vi "NodeMenuSelection.vi"(8 "error in (no error)":errorcluster, 9 "Item Path in":string, 10 "Menu Path in":string, 11 "xceRootNode in":refnum<class "xceRootNode.lvclass">) -> (0 "error out":errorcluster, 1 "Item Path out":string, 2 "Menu Path out":string, 3 "xceRootNode out":refnum<class "xceRootNode.lvclass">)   [LabVIEW 2013, in "xceRootNode.lvclass"]
doc: "Determines the action that must be performed based on the users tree control menu selection."
uses:
  xceRootNode.lvclass
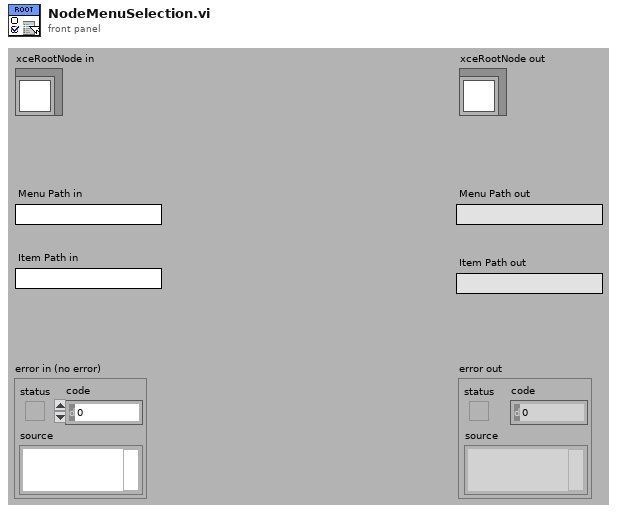
[diagram p1: front panel]
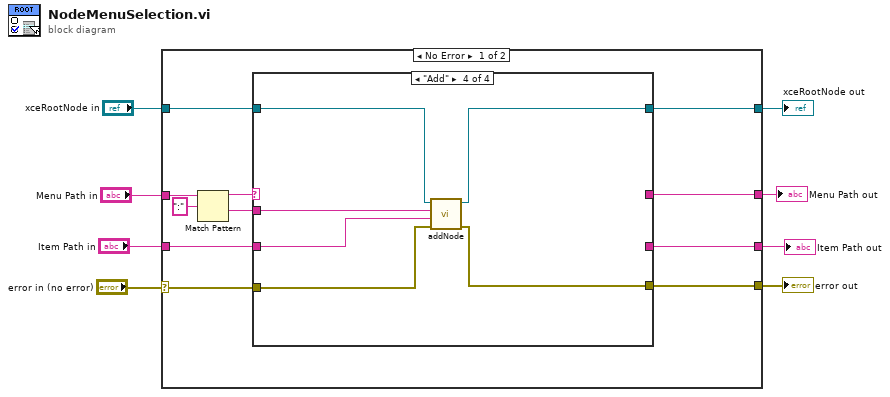
[diagram p0: block diagram]
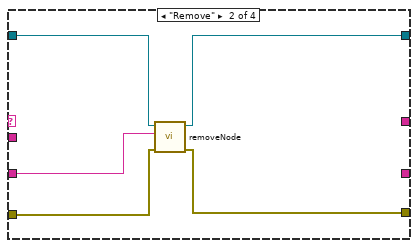
[diagram p3: hidden frame]
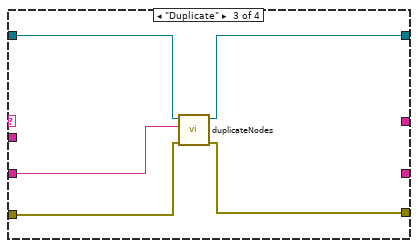
[diagram p4: hidden frame]
diagram:
  n1 = case shown="No Error" "error in (no error)" {
    selector: "error in (no error)" -> [w14 w41]
    tunnel: [w13 w41] -> w7
    tunnel: [w18 w40] -> w5
    tunnel: "xceRootNode in" -> [w19 w40]
    tunnel: "Menu Path in" -> [w12 _]
    tunnel: "Item Path in" -> [w17 _]
    tunnel: [w16 _] -> w2
    tunnel: [w15 _] -> w1
    frame No Error {
      n2 = Match Pattern(string=w12, regular expression=":") -> (before substring=w10:string, after substring=w9:string)  [unwired: 1 in, 2 out]
      n3 = case shown="\"Add\"" w10 {
        selector: w10 -> [w23 _ _ _]
        tunnel: w19 -> [w21 w28 w33 w39]
        tunnel: [w21 w27 w32 w38] -> w18
        tunnel: w17 -> [w22 w26 w31 w34]
        tunnel: [w23 _ _ _] -> w16
        tunnel: [w22 _ _ _] -> w15
        tunnel: w14 -> [w20 w25 w30 w36]
        tunnel: [w20 w24 w29 w35] -> w13
        tunnel: w9 -> [_ _ _ w37]
        frame "", Default {
        }
        frame "Remove" {
          n4 = call "removeNode.vi"("error in (no error)"=w25, "Node Path"=w26, "xceRootNode in"=w28) -> ("error out"=w24:errorcluster, "xceRootNode out"=w27:refnum<class "xceRootNode.lvclass">)  [unwired: 7 in]
        }
        frame "Duplicate" {
          n5 = call "duplicateNodes.vi"("error in (no error)"=w30, "Node Path"=w31, "xceRootNode in"=w33) -> ("error out"=w29:errorcluster, "xceRootNode out"=w32:refnum<class "xceRootNode.lvclass">)  [unwired: 7 in]
        }
        frame "Add" {
          n6 = call "addNode.vi"("error in (no error)"=w36, "superNode Path"=w34, "Data Class"=w37, "xceRootNode in"=w39) -> ("error out"=w35:errorcluster, "xceRootNode out"=w38:refnum<class "xceRootNode.lvclass">)  [unwired: 6 in]
        }
      }
    }
    frame Error {
    }
  }
  "error out" <- w7
  "xceRootNode out" <- w5
  "Item Path out" <- w1
  "Menu Path out" <- w2
